vi "Handle Request.vi"(7 "Processing In":refnum<class "Processing.lvclass">, 11 "Caching Request in":refnum<class "Caching Request.lvclass">) -> (0 "error out":errorcluster, 5 "Processing":refnum<class "Processing.lvclass">)   [LabVIEW 2023, in "HTTP Server.lvlib" / "Caching Request.lvclass"]
uses:
  Caching Request.lvclass
  Processing/Processing.lvclass
  Caching/Caching.lvclass
  C:/dev/volatus/mts-impulse/libs/lv-http-server/HTTP Server/Service/Service.lvclass
  Processing/Processing.lvclass/Processing.ctl
  lv-http-util/HTTP Utils/Request/Request.lvclass/Request.ctl
  lv-uri/URI/URI/URI.lvclass/URI.ctl
  lv-http-util/HTTP Utils/Request/Get Target URI.vi
  lv-uri/URI/URI/Path String.vi
  lv-http-util/HTTP Utils/HTTP Utils.lvlib
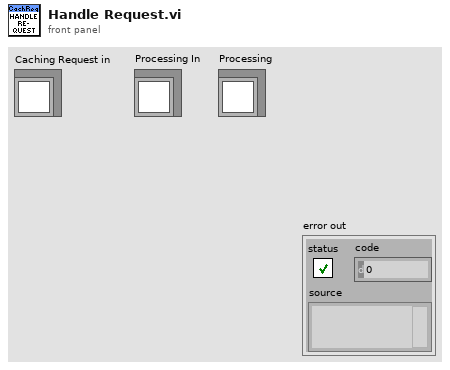
[diagram p1: front panel]
types:
  T1 = typedef "HTTP Server.lvlib/Request Cache Type.ctl" = enum16{"None", "Modified", "ETag", "Expires"}
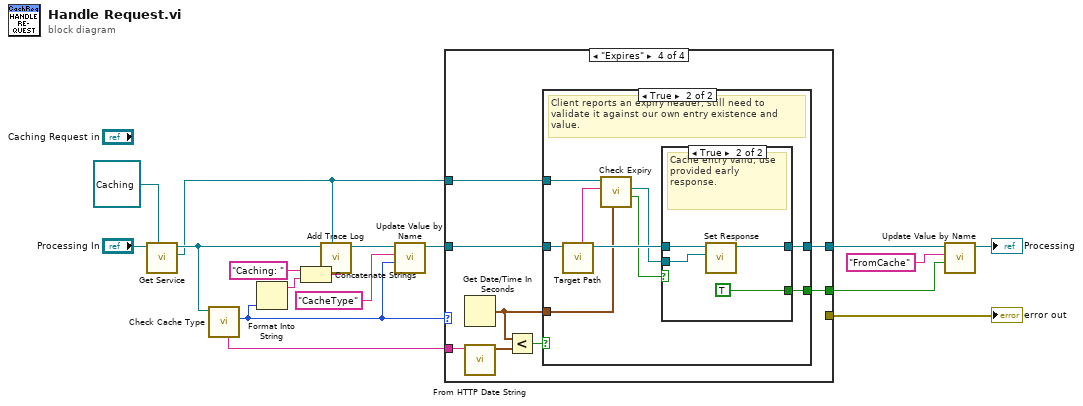
[diagram p0: block diagram]
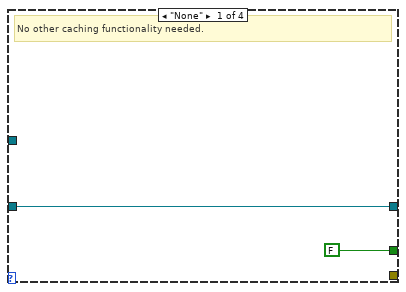
[diagram p2: hidden frame]
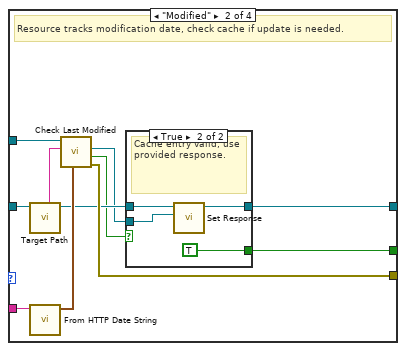
[diagram p3: hidden frame]
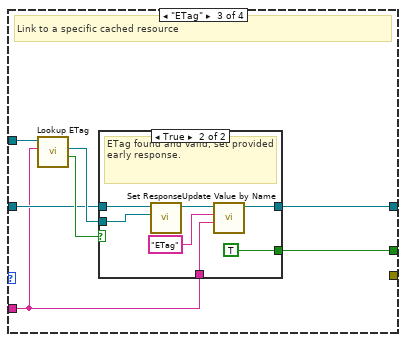
[diagram p5: hidden frame]
diagram:
  n1 = call "Get Service.vi"("Service Type"=refnum<class "Caching.lvclass"> refnum ("HTTP Server.lvlib:Caching.lvclass"), "Processing in"="Processing In") -> ("Service"=w10:refnum<class "Caching.lvclass">, "Processing out"=w11:refnum<class "Processing.lvclass">)  [unwired: 7 in, 1 out]
  n2 = call "Check Cache Type.vi"("Processing In"=w11) -> ("Request Cache Type"=w2:T1, "Value"=w14:string)  [unwired: 8 in, 1 out]
  n3 = Format Into String(w2) -> (resulting string=w17:string)  [unwired: 3 in, 1 out]
  n4 = Concatenate Strings("Caching: " ("string"), w17) -> (w16:string)
  n5 = call "Add Trace Log.vi"("Info"=w16, "LabVIEW Object"=w10, "Processing in"=w11) -> ("Processing out"=w8:refnum<class "Processing.lvclass">)  [unwired: 7 in, 1 out]
  n6 = call "Update Value by Name.vi"("Value"=w2, "Name"="CacheType" ("Name / Service / Object"), "Processing in"=w8) -> ("Processing out"=w9:refnum<class "Processing.lvclass">)  [unwired: 7 in, 1 out]
  n7 = case shown="\"Expires\"" w2 {
    tunnel: w10 -> [_ w28 w42 w55]
    tunnel: w9 -> [w19 w27 w38 w56]
    tunnel: [w19 w21 w39 w53] -> w6
    tunnel: w14 -> [_ w29 w37 w58]
    tunnel: [_ w30 _ _] -> w13
    tunnel: [FALSE w20 w36 w51] -> w1
    frame "None" {
      # "No other caching functionality needed."
    }
    frame "Modified" {
      # "Resource tracks modification date, check cache if update is needed."
      n8 = call "Target Path.vi"("Processing in"=w27) -> ("Processing out"=w24:refnum<class "Processing.lvclass">, "Target Path"=w26:string)  [unwired: 9 in]
      n9 = call "From HTTP Date String.vi"("HTTP Date String"=w29) -> ("Time Stamp"=w25:timestamp)  [unwired: 10 in]
      n10 = call "Check Last Modified.vi"("Last-Modified"=w25, "Target Path"=w26, "Caching in"=w28) -> ("error out"=w30:errorcluster, "From Cache?"=w22:bool, "Response"=w23:refnum<class "Response.lvclass">)  [unwired: 5 in, 1 out]
      n11 = case shown="True" w22 {
        tunnel: w24 -> [w31 w35]
        tunnel: w23 -> [_ w34]
        tunnel: [w31 w33] -> w21
        tunnel: [_ TRUE] -> w20
        frame False {
          # "Entry not found or stale. Follow normal processing flow."
        }
        frame True {
          # "Cache entry valid, use provided response."
          n12 = call "Set Response.vi"("Response"=w34, "Processing in"=w35) -> ("Processing out"=w33:refnum<class "Processing.lvclass">)  [unwired: 9 in]
        }
      }
    }
    frame "ETag" {
      # "Link to a specific cached resource"
      n13 = call "Lookup ETag.vi"("ETag"=w37, "Caching in"=w42) -> ("From Cache?"=w41:bool, "Response"=w40:refnum<class "Response.lvclass">)  [unwired: 6 in, 2 out]
      n14 = case shown="True" w41 {
        tunnel: w38 -> [w43 w50]
        tunnel: w40 -> [_ w49]
        tunnel: [w43 w45] -> w39
        tunnel: w37 -> [_ w46]
        tunnel: [_ TRUE] -> w36
        frame False {
          # "ETag not found or invalid, follow normal processing flow."
        }
        frame True {
          # "ETag found and valid, set provided early response."
          n15 = call "Set Response.vi"("Response"=w49, "Processing in"=w50) -> ("Processing out"=w48:refnum<class "Processing.lvclass">)  [unwired: 9 in]
          n16 = call "Update Value by Name.vi"("Value"=w46, "Name"="ETag" ("Name / Service / Object"), "Processing in"=w48) -> ("Processing out"=w45:refnum<class "Processing.lvclass">)  [unwired: 7 in, 1 out]
        }
      }
    }
    frame "Expires" {
      n17 = Get Date/Time In Seconds() -> (seconds since 1Jan1904=w52:timestamp)
      n18 = call "From HTTP Date String.vi"("HTTP Date String"=w58) -> ("Time Stamp"=w54:timestamp)  [unwired: 10 in]
      n19 = Less?(x=w52, y=w54) -> (x < y?=w57:bool)
      n20 = case shown="True" w57 {
        tunnel: w56 -> [w59 w67]
        tunnel: w55 -> [_ w68]
        tunnel: [w59 w62] -> w53
        tunnel: w52 -> [_ w61]
        tunnel: [_ w60] -> w51
        frame False {
          # "Client header already expired, follow normal processing."
        }
        frame True {
          # "Client reports an expiry header, still need to validate it against our own entry existence and value."
          n21 = call "Target Path.vi"("Processing in"=w67) -> ("Processing out"=w65:refnum<class "Processing.lvclass">, "Target Path"=w66:string)  [unwired: 9 in]
          n22 = call "Check Expiry.vi"("Now"=w61, "Target Path"=w66, "Caching in"=w68) -> ("From Cache?"=w64:bool, "Response"=w63:refnum<class "Response.lvclass">)  [unwired: 5 in, 2 out]
          n23 = case shown="True" w64 {
            tunnel: w65 -> [w69 w73]
            tunnel: w63 -> [_ w72]
            tunnel: [w69 w70] -> w62
            tunnel: [_ TRUE] -> w60
            frame False {
              # "Entry not found or stale. Follow normal processing flow."
            }
            frame True {
              # "Cache entry valid, use provided early response."
              n24 = call "Set Response.vi"("Response"=w72, "Processing in"=w73) -> ("Processing out"=w70:refnum<class "Processing.lvclass">)  [unwired: 9 in]
            }
          }
        }
      }
    }
  }
  "error out" <- w13
  n25 = call "Update Value by Name.vi"("Value"=w1, "Name"="FromCache" ("Name / Service / Object"), "Processing in"=w6) -> ("Processing out"=→"Processing":refnum<class "Processing.lvclass">)  [unwired: 7 in, 1 out]
